vi "Draw.vi"(8 "error in (no error)":errorcluster, 10 "picture in (empty picture)":picture, 11 "Ellipse in":refnum<class "Ellipse.lvclass">) -> (0 "error out":errorcluster, 2 "picture out":picture, 3 "Ellipse out":refnum<class "Ellipse.lvclass">)   [LabVIEW 2018, in "Ellipse.lvclass"]
doc: "Draw an ellipse"
uses:
  Ellipse.lvclass
  Ellipse.lvclass/Ellipse.ctl
panel:
  # "expressionflow.com"
  # "Copyright (c) 2008 Tomi Maila. All rights reserved."
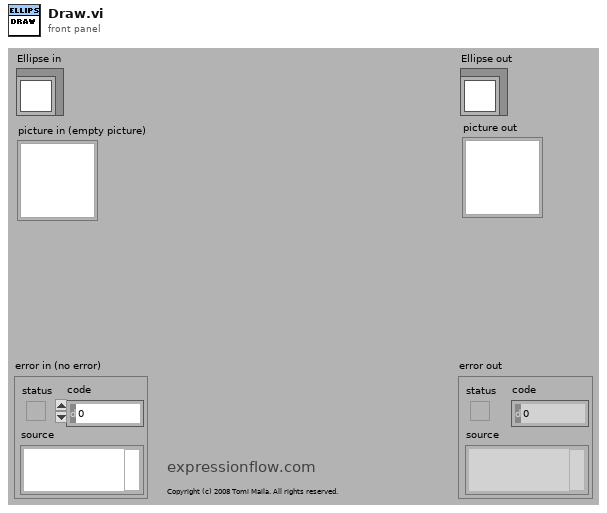
[diagram p1: front panel]
types:
  T1 = cluster{"Width":u16, "Style":enum32{"Solid", "Dash", "Dot", "DashDot", "DashDotDot"}}
  T2 = cluster{"left":i16, "top":i16, "right":i16, "bottom":i16}
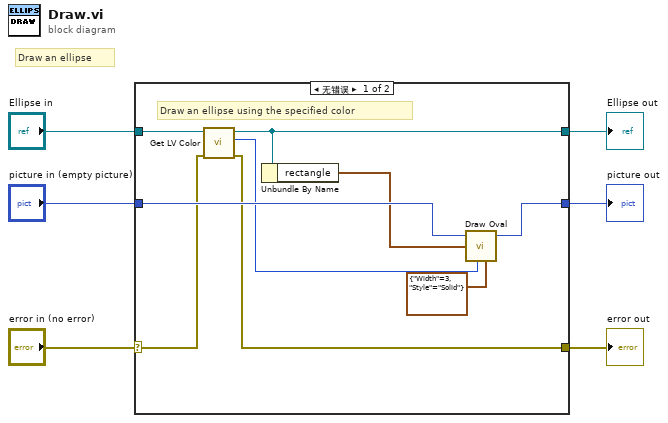
[diagram p0: block diagram]
diagram:
  # "Draw an ellipse"
  n1 = case shown="无错误" "error in (no error)" {
    selector: "error in (no error)" -> [w9 w17]
    tunnel: [w14 w18] -> w5
    tunnel: "picture in (empty picture)" -> [w15 w18]
    tunnel: [w12 w17] -> w3
    tunnel: [w7 w16] -> w2
    tunnel: "Ellipse in" -> [w10 w16]
    frame No Error {
      # "Draw an ellipse using the specified color"
      n2 = call-dynamic "Get LV Color.vi"("error in (no error)"=w9, "Graphics Object.lvclass in"=w10) -> ("error out"=w12:errorcluster, "Color"=w13:u32, "Graphics Object.lvclass out"=w7:refnum<class "Ellipse.lvclass">)  [unwired: 7 in]
      n3 = Unbundle By Name(w7) -> ("rectangle"=w11:T2)
      n4 = call <vilib>:"Draw Oval.vi"("picture"=w15, "rect"=w11, "color(black)"=w13, "pen"=T1 {"Width"=3, "Style"=enum."Solid"}) -> ("new picture"=w14:picture)  [unwired: 5 in]
    }
    frame Error {
    }
  }
  "error out" <- w3
  "Ellipse out" <- w2
  "picture out" <- w5
